vi "Lookup Query.vi"(10 "Name":string, 11 "URI in":refnum<class "URI.lvclass">) -> (1 "Found":bool, 2 "Value":string, 3 "URI out":refnum<class "URI.lvclass">)   [LabVIEW 2020, in "URI.lvlib" / "URI.lvclass"]
uses:
  URI.lvclass
  URI.lvclass/URI.ctl
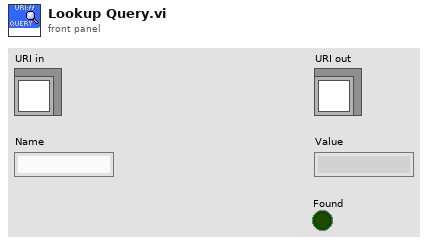
[diagram p1: front panel]
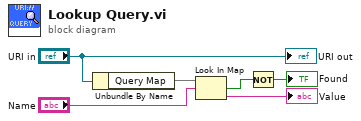
[diagram p0: block diagram]
diagram:
  n1 = Unbundle By Name("URI in") -> ("Query Map"=w5:map{string, string})
  n2 = Look In Map(map=w5, key="Name") -> (key not found?=w2:bool, value=→"Value":string)  [unwired: 1 in]
  n3 = Not(x=w2) -> (.not. x?=→"Found":bool)
  "URI out" <- "URI in"
